vi "SPC_get_photon.vi"(6 "Stream Handle":i16, 8 "Error In":errorcluster, 10 "Module No":i16, 11 "DLL Path":path) -> (0 "Error Out":errorcluster, 2 "Module No":i16, 3 "DLL Path":path, 4 "Stream Handle":i16, 5 "PhotInfo":T1 {"Flags" max=3 format="%016b"; "Routing channel" step=1; "Micro time value" step=1; "Macro time clocks high" step=1; "Macro time clocks low" step=1})   [LabVIEW 2023]
doc: "The procedure can be used in a loop to extract subsequent photons from the opened photons stream defined by handle 'stream_hndl'. It accepts only streams of spc files.\nTo extract photons from buffered photons streams SPC_get_photons_from_stream function can be used. \nThe procedure fills 'phot_info' structure with the information of the photon extracted from the current stream position. After extracting procedure updates internal stream structures. \nIf needed, it opens and read data from the next stream file. \nUse SPC_get_phot_stream_info function to get current stream state. \nProcedure returns error, if 'stream_hndl' is not the handle of the stream opened using SPC_init_phot_stream function.\nPhotInfo structure is defined in the spcm_def.h file.\n\ninfo@becker-hickl.com"
uses:
  SPC_Controls/SPC_PhotInfo.ctl
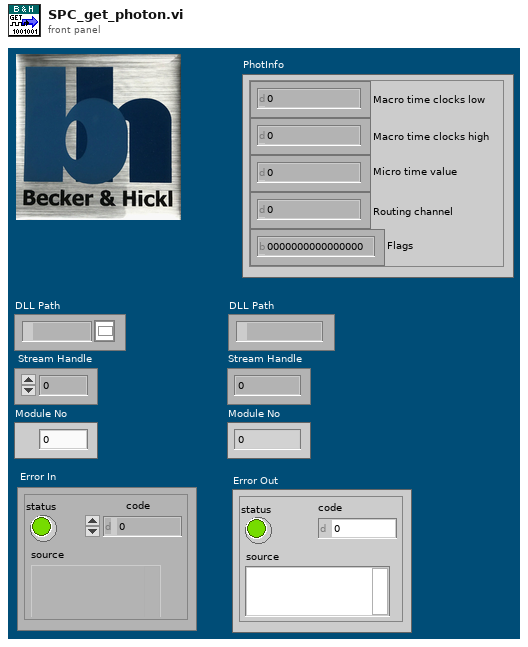
[diagram p1: front panel]
types:
  T1 = typedef "SPC_PhotInfo.ctl" = cluster{"Macro time clocks low":u32, "Macro time clocks high":u32, "Micro time value":u16, "Routing channel":u16, "Flags":u16}
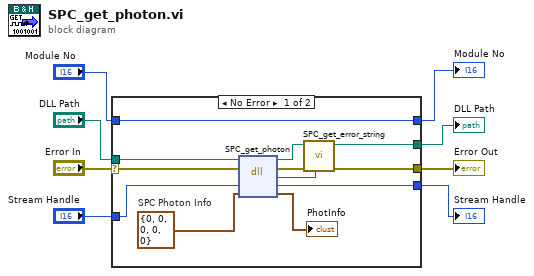
[diagram p0: block diagram]
diagram:
  n1 = case shown="No Error" "Error In" {
    selector: "Error In" -> [w20 w24]
    tunnel: [w18 w24] -> w7
    tunnel: [w12 w23] -> w6
    tunnel: "DLL Path" -> [w17 w23]
    tunnel: "Stream Handle" -> [w15 w22]
    tunnel: [w14 w22] -> w3
    tunnel: [w11 w21] -> w2
    tunnel: "Module No" -> [w11 w21]
    frame No Error {
      w10 = T1 {"Macro time clocks low"=0, "Macro time clocks high"=0, "Micro time value"=0, "Routing channel"=0, "Flags"=0}  # SPC Photon Info
      n2 = dll-call lib="D:/spcm/lib/lab_view/lv10.0/spcm32.dll" fn="SPC_get_photon"(path in=w17, error in=w20, "stream_hndl"=w15, "phot_info"=w10) -> (path out=w13:path, error out=w19:errorcluster, "return type"=w16:i16, "stream_hndl"=w14:i16, "phot_info"=→"PhotInfo":T1)  [unwired: 1 in]
      n3 = call "SPC_get_error_string.vi"("ErrorID"=w16, "Error In"=w19, "DLL Path"=w13) -> ("Error Out"=w18:errorcluster, "DLL Path"=w12:path)  [unwired: 6 in, 1 out]
    }
    frame Error {
    }
  }
  "DLL Path" <- w6
  "Error Out" <- w7
  "Stream Handle" <- w3
  "Module No" <- w2
